vi "Three-Motor-Speed-Control.vi"(7 "Reset":bool, 8 "Error In":errorcluster, 11 "速度(秒/度)":dbl[](array[numeric])) -> (0 "Error Out":errorcluster)   [LabVIEW 2019]
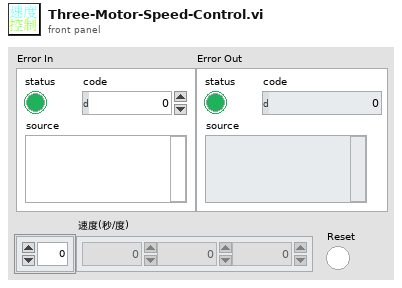
[diagram p1: front panel]
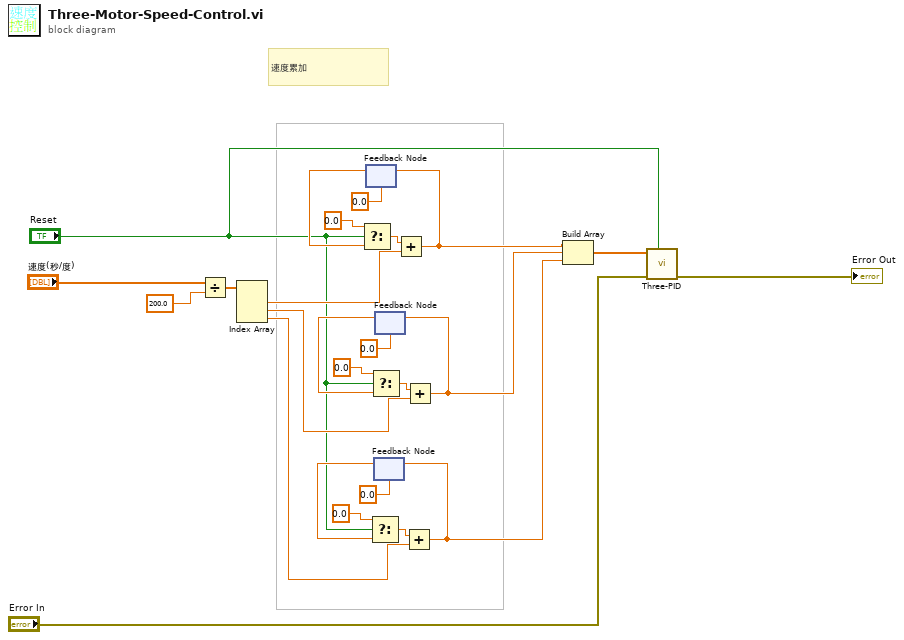
[diagram p0: block diagram]
diagram:
  # "速度累加"
  n1 = Divide(x="速度(秒/度)", y=200.0) -> (x/y=w22:dbl[])
  n2 = Index Array(array=w22) -> (element #1=w21:dbl, element #2=w8:dbl, element #3=w7:dbl)  [unwired: 3 in]
  n3 = feedback #1(0.0) -> (w19:dbl)
  n4 = Select(t=0.0, s="Reset", f=w19) -> (s? t:f=w20:dbl)
  n5 = feedback #2(0.0) -> (w11:dbl)
  n6 = Select(t=0.0, s="Reset", f=w11) -> (s? t:f=w12:dbl)
  n7 = feedback #3(0.0) -> (w15:dbl)
  n8 = Select(t=0.0, s="Reset", f=w15) -> (s? t:f=w16:dbl)
  n9 = Add(x=w20, y=w21) -> (x+y=w6:dbl)
  n10 = feedback-in #1(w6) -> ()
  n11 = Add(x=w12, y=w7) -> (x+y=w4:dbl)
  n12 = feedback-in #2(w4) -> ()
  n13 = Add(x=w16, y=w8) -> (x+y=w5:dbl)
  n14 = feedback-in #3(w5) -> ()
  n15 = Build Array(w6, w5, w4) -> (w3:dbl[])
  n16 = call "Three-PID.vi"("Reset"="Reset", "Error In"="Error In", "目標角度"=w3) -> ("Error Out"=→"Error Out":errorcluster)  [unwired: 8 in]
